vi "Read Bytes.vi"(8 "error in (no error)":errorcluster, 11 "Multipart Parser in":refnum<class "Multipart Parser.lvclass">) -> (0 "error out":errorcluster, 2 "Value":string, 3 "Multipart Parser out":refnum<class "Multipart Parser.lvclass">, 4 "Boundary":bool, 5 "Last":bool)   [LabVIEW 2020, in "HTTP Utils.lvlib" / "Multipart Parser.lvclass"]
uses:
  Multipart Parser.lvclass
  Multipart Parser.lvclass/Multipart Parser.ctl
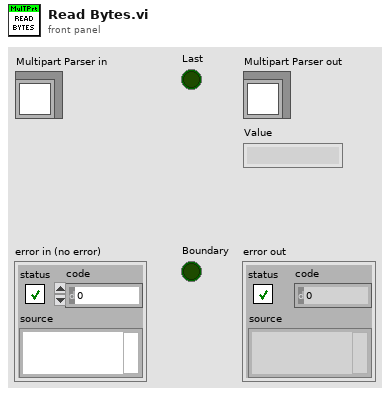
[diagram p1: front panel]
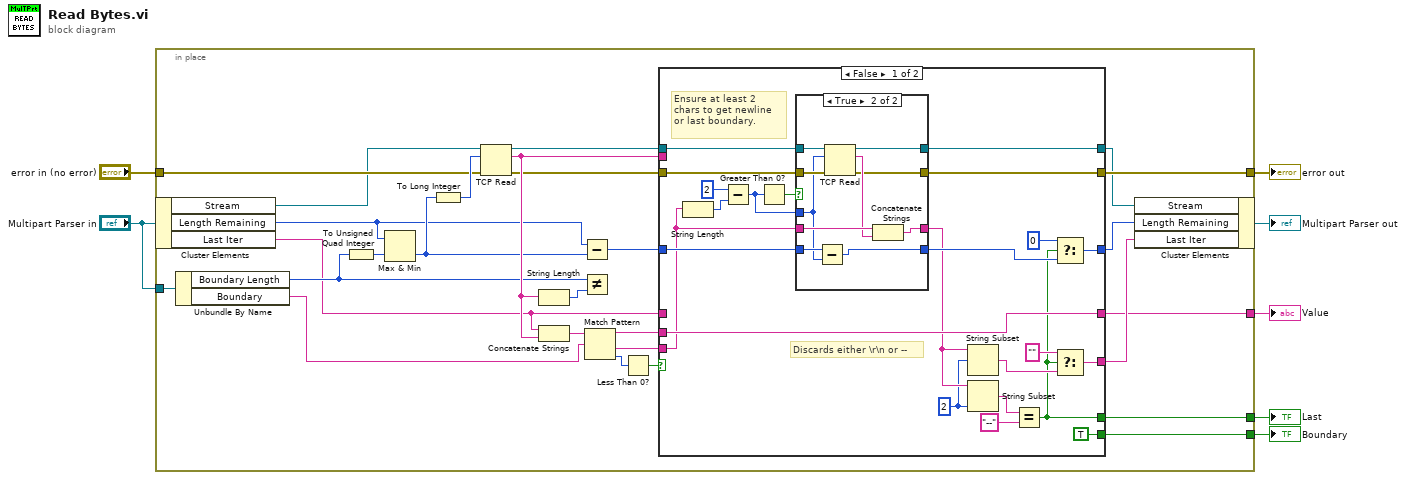
[diagram p0: block diagram]
diagram:
  n1 = in-place {
    in-place-border: "error in (no error)" -> [w21]
    in-place-border: [w17] -> w6
    in-place-border: "Multipart Parser in" -> [w14]
    in-place-border: [w12] -> w2
    in-place-border: [w11] -> w4
    in-place-border: [w10] -> w3
    n2 = in-place-cluster #1("Multipart Parser in") -> ("Stream"=w20:refnum<k5>, "Length Remaining"=w19:u64, "Last Iter"=w8:string)
    n3 = Unbundle By Name(w14) -> ("Boundary Length"=w9:i32, "Boundary"=w13:string)
    n4 = To Unsigned Quad Integer(1:w9) -> (0:w32:u64)
    n5 = Max & Min(x=w19, y=w32) -> (min(x,y)=w22:u64)  [unwired: 1 out]
    n6 = To Long Integer(number=w22) -> (32bit integer=w25:i32)
    n7 = TCP Read(connection ID=w20, bytes to read=w25, error in (no error)=w21) -> (connection ID out=w24:refnum<k5>, data out=w29:string, error out=w23:errorcluster)  [unwired: 2 in]
    n8 = String Length(string=w29) -> (length=w28:i32)
    n9 = Concatenate Strings(w8, w29) -> (w34:string)
    n10 = Subtract(x=w19, y=w22) -> (x-y=w26:u64)
    n11 = Not Equal?(x=w9, y=w28) -> ()  [unwired: 1 out]
    n12 = Match Pattern(string=w34, regular expression=w13) -> (before substring=w27:string, after substring=w31:string, offset past match=w33:i32)  [unwired: 1 in, 1 out]
    n13 = Less Than 0?(x=w33) -> (x < 0?=w30:bool)
    n14 = case shown="False" w30 {
      tunnel: w31 -> [w43 _]
      tunnel: w29 -> [_ w76]
      tunnel: w8 -> [_ w75]
      tunnel: [w54 w76] -> w15
      tunnel: [w51 w75] -> w12
      tunnel: w27 -> [w51 _]
      tunnel: w26 -> [w45 w74]
      tunnel: [w52 w74] -> w18
      tunnel: w24 -> [w47 w73]
      tunnel: w23 -> [w46 w72]
      tunnel: [w41 w73] -> w16
      tunnel: [w40 w72] -> w17
      tunnel: [TRUE _] -> w11
      tunnel: [w36 _] -> w10
      frame False {
        w37 = 2 ("length (rest)")
        # "Discards either \\r\\n or --"
        # "Ensure at least 2 chars to get newline or last boundary."
        n15 = String Length(string=w43) -> (length=w50:i32)
        n16 = Subtract(x=2, y=w50) -> (x-y=w44:i32)
        n17 = Greater Than 0?(x=w44) -> (x > 0?=w48:bool)
        n18 = case shown="True" w48 {
          tunnel: w47 -> [w59 w71]
          tunnel: w46 -> [w58 w70]
          tunnel: w45 -> [w61 w67]
          tunnel: w44 -> [_ w66]
          tunnel: w43 -> [w60 w69]
          tunnel: [w61 w64] -> w42
          tunnel: [w60 w65] -> w38
          tunnel: [w59 w63] -> w41
          tunnel: [w58 w62] -> w40
          frame False {
          }
          frame True {
            n19 = Subtract(x=w67, y=w66) -> (x-y=w64:u64)
            n20 = TCP Read(connection ID=w71, bytes to read=w66, error in (no error)=w70) -> (connection ID out=w63:refnum<k5>, data out=w68:string, error out=w62:errorcluster)  [unwired: 2 in]
            n21 = Concatenate Strings(w69, w68) -> (w65:string)
          }
        }
        n22 = String Subset(string=w38, offset (0)=w37) -> (substring=w39:string)  [unwired: 1 in]
        n23 = String Subset(string=w38, length (rest)=w37) -> (substring=w57:string)  [unwired: 1 in]
        n24 = Equal?(x=w57, y="--") -> (x = y?=w36:bool)
        n25 = Select(t=u64 0, s=w36, f=w42) -> (s? t:f=w52:u64)
        n26 = Select(t="", s=w36, f=w39) -> (s? t:f=w54:string)
      }
      frame True {
      }
    }
    n27 = in-place-cluster #1("Stream"=w16, "Length Remaining"=w18, "Last Iter"=w15) -> (→"Multipart Parser out":refnum<class "Multipart Parser.lvclass">)
  }
  "error out" <- w6
  "Boundary" <- w4
  "Value" <- w2
  "Last" <- w3
